vi "ManageWebSocket.vi"(8 "error in":errorcluster, 11 "webSocketCluster_typeDef in":T1) -> (0 "error out":errorcluster)   [LabVIEW 2024]
uses:
  Control/webSocketCluster_typeDef.ctl
  Control/webSocket_globalVar_states.ctl
  <vilib>/MediaMongrels Ltd/WebSockets/Sockets/VISA TCP Socket/VISA TCP.lvclass
  C:/Program Files/National Instruments/LabVIEW 2024/vi.lib/MediaMongrels Ltd/WebSockets/Sockets/Socket/Socket.lvclass
  GlobalVars/webSocketVars.vi
  <vilib>/MediaMongrels Ltd/WebSockets/WebSockets/WebSocket Server/WebSocket Server.lvclass
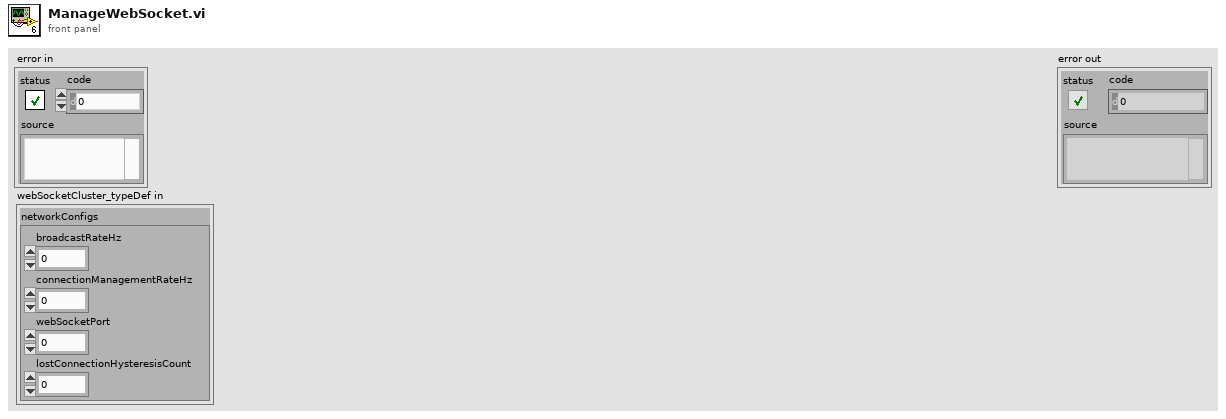
[diagram p1: front panel]
types:
  T1 = typedef "webSocketCluster_typeDef.ctl" = cluster{"networkConfigs":cluster{"broadcastRateHz":i32, "connectionManagementRateHz":i32, "webSocketPort":i32, "lostConnectionHysteresisCount":i32}}
  T2 = typedef "webSocket_globalVar_states.ctl" = enum16{"starting", "streaming", "close", "fault"}
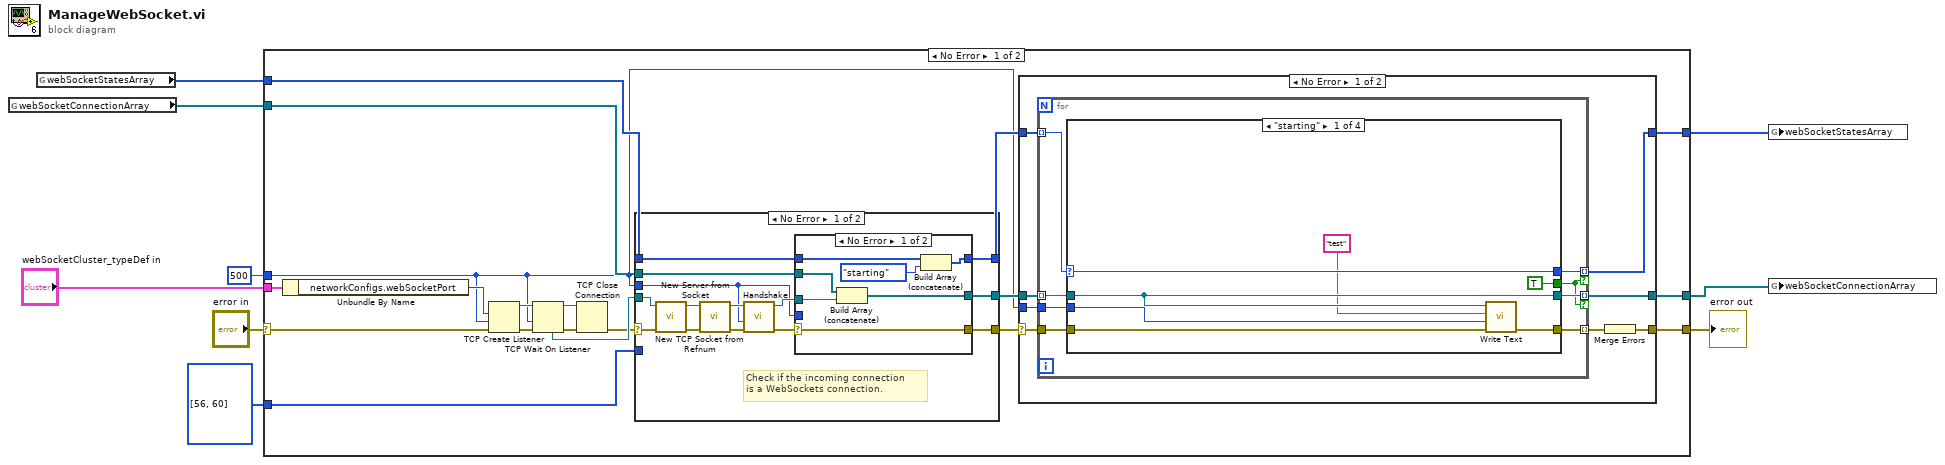
[diagram p0: block diagram]
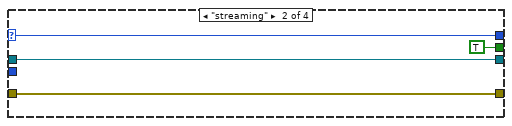
[diagram p2: hidden frame]
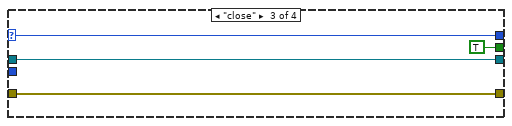
[diagram p3: hidden frame]
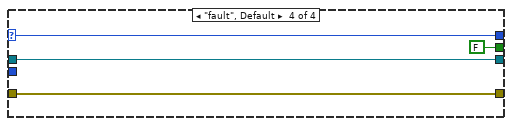
[diagram p4: hidden frame]
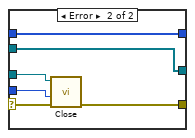
[diagram p6: hidden frame]
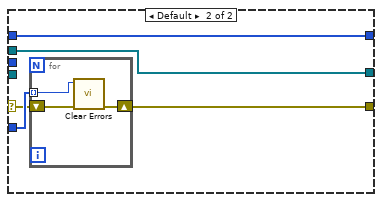
[diagram p7: hidden frame]
diagram:
  n1 = global read "webSocketVars.vi" "webSocketConnectionArray"() -> (w5:refnum<class "WebSocket Server.lvclass">[])
  n2 = global read "webSocketVars.vi" "webSocketStatesArray"() -> (w4:T2[])
  n3 = case shown="No Error" "error in" {
    selector: "error in" -> [w23 w104]
    tunnel: [w16 w104] -> w8
    tunnel: "webSocketCluster_typeDef in" -> [w28 _]
    tunnel: i32[] [56, 60] -> [w27 _]
    tunnel: w5 -> [w19 w103]
    tunnel: w4 -> [w18 w102]
    tunnel: [w15 w103] -> w3
    tunnel: [w12 w102] -> w2
    tunnel: 500 ("timeout ms (25000)") -> [w10 _]
    frame No Error {
      n4 = Unbundle By Name(w28) -> ("networkConfigs.webSocketPort"=w11:i32)
      n5 = TCP Create Listener(8:w23, 9:w10, 10:w11) -> (0:w25:errorcluster, 3:w26:refnum<k5>)  [unwired: 2 in, 1 out]
      n6 = TCP Wait On Listener(8:w25, 9:w10, 11:w26) -> (0:w22:errorcluster, 3:w20:refnum<k5>, 4:w24:refnum<k5>)  [unwired: 1 in, 2 out]
      n7 = TCP Close Connection(connection ID=w20, error in (no error)=w22) -> (error out=w21:errorcluster)  [unwired: 1 in, 1 out]
      n8 = case shown="No Error" w21 {
        selector: w21 -> [w77 w96]
        tunnel: w10 -> [w71 _]
        tunnel: [w72 w98] -> w17
        tunnel: w27 -> [_ w97]
        tunnel: w24 -> [w74 _]
        tunnel: w19 -> [w70 w95]
        tunnel: w18 -> [w69 w94]
        tunnel: [w68 w95] -> w14
        tunnel: [w67 w94] -> w13
        frame No Error {
          # "Check if the incoming connection\nis a WebSockets connection."
          n9 = call <vilib>:"New TCP Socket from Refnum.vi"("error in (no error)"=w77, "TCP Network Connection Refnum"=w74) -> ("error out"=w76:errorcluster, "VISA TCP out"=w75:refnum<class "VISA TCP.lvclass">)  [unwired: 8 in]
          n10 = call <vilib>:"New Server from Socket.vi"("error in (no error)"=w76, "Socket"=w75) -> ("error out"=w79:errorcluster, "WebSocket Server out"=w80:refnum<class "WebSocket Server.lvclass">)  [unwired: 8 in]
          n11 = call-dynamic "Handshake.vi"("error in (no error)"=w79, "timeout ms (5000)"=w71, "WebSocket Connection in"=w80) -> ("error out"=w73:errorcluster, "WebSocket Connection out"=w78:refnum<class "WebSocket Server.lvclass">)  [unwired: 7 in]
          n12 = case shown="No Error" w73 {
            selector: w73 -> [w85 w91]
            tunnel: w78 -> [w87 w92]
            tunnel: [w85 w90] -> w72
            tunnel: w71 -> [_ w93]
            tunnel: w70 -> [w84 w89]
            tunnel: w69 -> [w83 w88]
            tunnel: [w82 w89] -> w68
            tunnel: [w81 w88] -> w67
            frame No Error {
              n13 = Build Array (concatenate)(w84, w87) -> (w82:refnum<class "WebSocket Server.lvclass">[])
              n14 = Build Array (concatenate)(w83, webSocket_globalVar_states."starting") -> (w81:T2[])
            }
            frame Error {
              n15 = call-dynamic "Close.vi"("error in (no error)"=w91, "timeout ms (5000)"=w93, "WebSocket in"=w92) -> ("error out"=w90:errorcluster)  [unwired: 8 in]
            }
          }
        }
        frame Default {
          n16 = for {
            shift-right: [w101] -> w98
            shift-left: w96 -> [w100]
            tunnel: w97 -> [w99] mode=indexing
            n17 = call <vilib>:"Clear Errors.vi"("error in (no error)"=w100, "specific error code to clear (0: all)"=w99) -> ("error out"=w101:errorcluster)  [unwired: 4 in, 1 out]
          }
        }
      }
      n18 = case shown="No Error" w17 {
        selector: w17 -> [w34 w66]
        tunnel: [w33 w66] -> w16
        tunnel: [w31 w65] -> w15
        tunnel: w14 -> [w35 w65]
        tunnel: w13 -> [w36 w64]
        tunnel: [w30 w64] -> w12
        tunnel: w10 -> [w29 _]
        frame No Error {
          n19 = for {
            tunnel: w36 -> [w44] mode=indexing
            tunnel: w35 -> [w43] mode=indexing
            tunnel: w34 -> [w42]
            tunnel: [w41] -> w32 mode=indexing
            tunnel: [w40] -> w31 mode=indexing if=w38
            tunnel: [w39] -> w30 mode=indexing if=w38
            tunnel: w29 -> [w37]
            n20 = case shown="\"starting\"" w44 {
              selector: w44 -> [w46 w55 w59 w62]
              tunnel: w43 -> [w48 w53 w57 w61]
              tunnel: w42 -> [w50 w52 w56 w63]
              tunnel: [w49 w52 w56 w63] -> w41
              tunnel: [w48 w53 w57 w61] -> w40
              tunnel: [w46 w55 w59 w62] -> w39
              tunnel: [TRUE TRUE TRUE FALSE] -> w38
              tunnel: w37 -> [w47 _ _ _]
              frame "starting" {
                n21 = call-dynamic "Write Text.vi"("error in (no error)"=w50, "timeout ms (5000)"=w47, "String Data"="test", "WebSocket in"=w48) -> ("error out"=w49:errorcluster)  [unwired: 6 in, 1 out]
              }
              frame "streaming" {
              }
              frame "close" {
              }
              frame "fault", Default {
              }
            }
          }
          n22 = Merge Errors(w32) -> (w33:errorcluster)
        }
        frame Error {
        }
      }
    }
    frame Error {
    }
  }
  "error out" <- w8
  n23 = global write "webSocketVars.vi" "webSocketStatesArray"(w2) -> ()
  n24 = global write "webSocketVars.vi" "webSocketConnectionArray"(w3) -> ()
